vi "Write Name.vi"(8 "error in (no error)":errorcluster, 10 "Name":string, 11 "Attribute in":refnum<class "Attribute.lvclass">) -> (0 "error out":errorcluster, 3 "Attribute out":refnum<class "Attribute.lvclass">)   [LabVIEW 2020, in "VILab.lvlib" / "Attribute.lvclass"]
uses:
  Attribute.lvclass
  Attribute.lvclass/Attribute.ctl
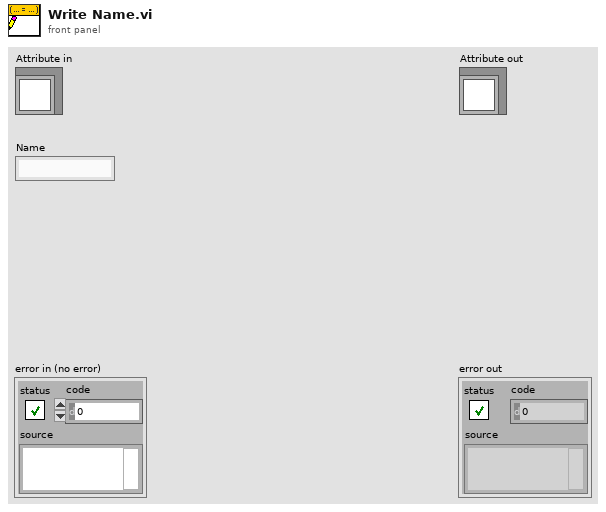
[diagram p1: front panel]
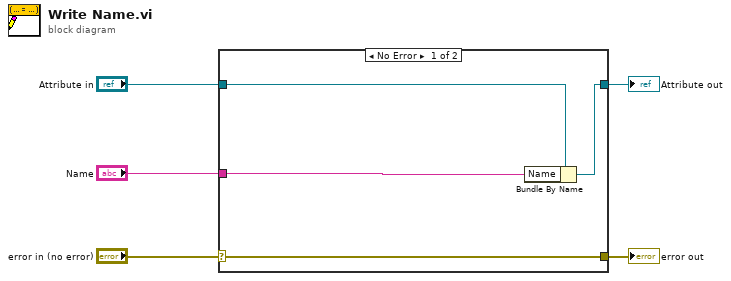
[diagram p0: block diagram]
diagram:
  n1 = case shown="No Error" "error in (no error)" {
    selector: "error in (no error)" -> [w9 w10]
    tunnel: [w9 w10] -> w4
    tunnel: [w7 w11] -> w2
    tunnel: "Attribute in" -> [w8 w11]
    tunnel: "Name" -> [w6 _]
    frame No Error {
      n2 = Bundle By Name(cluster=w8, "Name"=w6) -> (w7:refnum<class "Attribute.lvclass">)
    }
    frame Error {
    }
  }
  "error out" <- w4
  "Attribute out" <- w2
